vi "IMAQ FPGA Pixel Bus to FIFO U8x16.vi"(8 "Input Valid":bool=TRUE, 10 "Destination Image FIFO":refnum<k21>, 11 "Pixel Bus In":T1={"Pixel Data"=[0, 0, 0, 0, 0, 0, 0, 0, 0, 0, 0, 0, 0, 0, 0, 0], "DV"=[FALSE, FALSE, FALSE, FALSE, FALSE, FALSE, FALSE, FALSE, FALSE, FALSE, FALSE, FALSE, FALSE, FALSE, FALSE, FALSE], "EOL"=FALSE, "EOI"=FALSE, "Data Type"=enum."U8 x 16"}) -> (4 "Ready for Input":bool)   [LabVIEW 2020, in "NI_VDM_FPGA_Basics.lvlib"]
doc: "Writes valid Pixel Data in the Pixel Bus cluster to the specified FIFO. If the FIFO is full, the Ready for Input terminal returns FALSE during that cycle."
uses:
  <vilib>/visionFPGA/NI_VDM_FPGA_Basics.lvlib
  <vilib>/rvi/DataTransferAndStorage/Container/XNode/niFpgaContainer.xnode
  <vilib>/rvi/FIFO/Fifo_Resource/niFpgaFifoEmulationRefInMultiElement.vi
  <vilib>/visionFPGA/Controls/IMAQ FPGA Pixel Bus u8x16.ctl
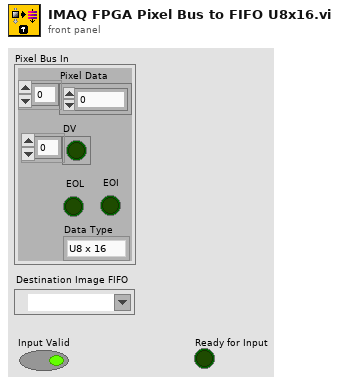
[diagram p1: front panel]
types:
  T1 = typedef "IMAQ FPGA Pixel Bus u8x16.ctl" = cluster{"Pixel Data":u8[], "DV":bool[], "EOL":bool, "EOI":bool, "Data Type":enum16{"U8 x 16"}}
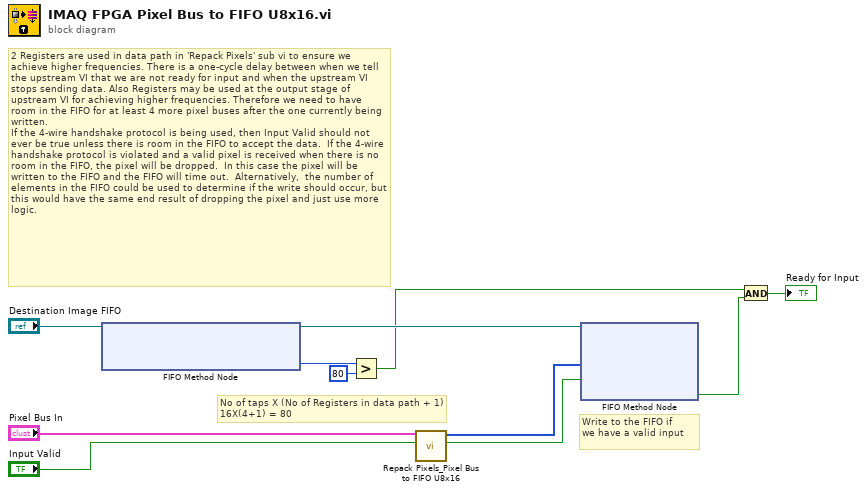
[diagram p0: block diagram]
diagram:
  # "No of taps X (No of Registers in data path + 1)\n16X(4+1) = 80"
  # "2 Registers are used in data path in 'Repack Pixels' sub vi to ensure we achieve higher frequencies. There is a one-cycle delay between when we tell the upstream VI that we are not ready for input and when the upstream VI stops sending data. Also Registers may be used at the output stage of upstream VI for achieving higher frequencies. Therefore we need to have room in the FIFO for at least 4 more pixel buses after the one currently being written. \nIf the 4-wire handshake protocol is being used, then Input Valid should not ever be true unless there is room in the FIFO to accept the data.  If the 4-wire handshake protocol is violated and a valid pixel is received when there is no room in the FIFO, the pixel will be dropped.  In this case the pixel will be written to the FIFO and the FIFO will time out.  Alternatively,  the number of elements in the FIFO could be used to determine if the write should occur, but this would have the same end result of dropping the pixel and just use more logic."
  # "Write to the FIFO if \nwe have a valid input"
  n1 = xnode ("FIFO Method Node")("FIFO In"="Destination Image FIFO") -> ("Number of Elements to Write"=w9:u32, "FIFO Out"=w10:refnum<k21>)
  n2 = Greater?(x=w9, y=u32 80) -> (0:w3:bool)
  n3 = call <vilib>:"Repack Pixels_Pixel Bus to FIFO U8x16.vi"("Input Valid"="Input Valid", "Pixel Bus In"="Pixel Bus In") -> ("Output Valid"=w4:bool, "Output Array"=w5:u8[])  [unwired: 8 in]
  n4 = xnode ("FIFO Method Node")("Element"=w5, "Input Valid"=w4, "FIFO In"=w10) -> ("Ready for Input"=w2:bool)  [unwired: 1 out]
  n5 = And(x=w3, y=w2) -> (x .and. y?=→"Ready for Input":bool)
